vi "Set Highlighted.vi"(8 "error in (no error)":errorcluster, 10 "Highlighted":bool, 11 "PlatformArrayPanel in":refnum<class "PlatformArrayPanel.lvclass">) -> (0 "error out":errorcluster, 3 "PlatformArrayPanel out":refnum<class "PlatformArrayPanel.lvclass">)   [LabVIEW 2020, in "PicoG-App.lvlib" / "PlatformArrayPanel.lvclass"]
uses:
  PlatformArrayPanel.lvclass
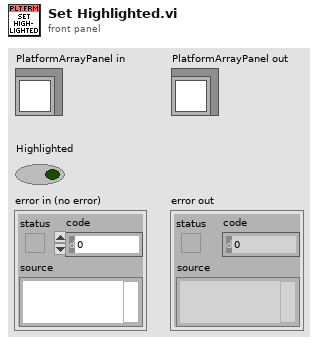
[diagram p1: front panel]
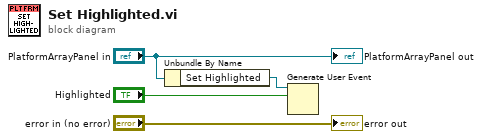
[diagram p0: block diagram]
diagram:
  n1 = Unbundle By Name("PlatformArrayPanel in") -> ("Set Highlighted"=w2:refnum<user-event>)
  n2 = Generate User Event(user event=w2, event data cluster="Highlighted") -> ()  [unwired: 2 in, 2 out]
  "error out" <- "error in (no error)"
  "PlatformArrayPanel out" <- "PlatformArrayPanel in"
